vi "I2C Open Channel.vi"(0 "handle":u32, 5 "index":u32, 11 "error in (no error)":errorcluster) -> (4 "handle out":u32, 15 "error out":errorcluster)   [LabVIEW 2017, in "libMPSSE.lvlib"]
doc: "FTDI_API FT_STATUS I2C_OpenChannel(uint32 index, FT_HANDLE *handle);"
uses:
  libMPSSE.lvlib
  libMPSSE-SPI-LabVIEW-master/libMPSSE.dll
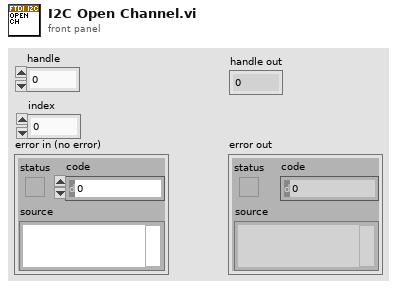
[diagram p1: front panel]
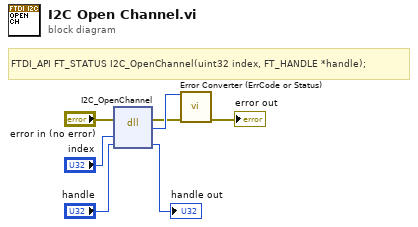
[diagram p0: block diagram]
diagram:
  # "FTDI_API FT_STATUS I2C_OpenChannel(uint32 index, FT_HANDLE *handle);"
  n1 = dll-call lib="\\\\Mac\\Home/Desktop/libMPSSE-SPI-LabVIEW-master/libMPSSE.dll" fn="I2C_OpenChannel"(error in="error in (no error)", "index"="index", "handle"="handle") -> (error out=w2:errorcluster, "return type"=w7:u32, "handle"=→"handle out":u32)  [unwired: 3 in, 1 out]
  n2 = call "Error Converter (ErrCode or Status).vi"("error code"=w7, "error in (no error)"=w2) -> ("error out"=→"error out":errorcluster)  [unwired: 13 in]
